vi "exercice5-4.vi"() -> ()   [LabVIEW 2013]
panel:
  out "cluster de sortie":cluster{"Nom de l'essai":string, dbl[]}
  in  "Cluster":T1
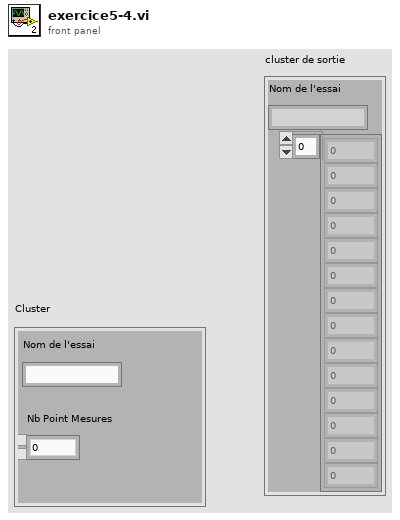
[diagram p1: front panel]
types:
  T1 = cluster{"Nom de l'essai":string, "Nb Point Mesures ":dbl}
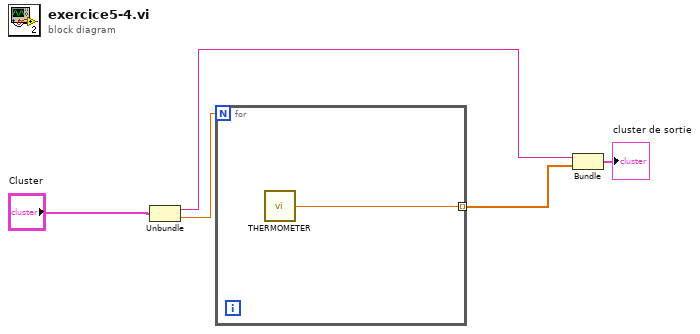
[diagram p0: block diagram]
diagram:
  n1 = Unbundle("Cluster") -> ("Nom de l'essai"=w2:string, "Nb Point Mesures"=w4:dbl)
  n2 = for {
    N: w4 -> [_]
    tunnel: [w6] -> w3 mode=indexing
    n3 = call "THERMOMETER.vi"() -> ("temeperature"=w6:dbl)  [unwired: 1 in]
  }
  n4 = Bundle("Nom de l'essai"=w2, w3) -> (→"cluster de sortie":cluster{"Nom de l'essai":string, dbl[]})  [unwired: 1 in]
